vi "Update Contingency (SubVI).vi"(0 "array 1":i32[](array[numeric]), 1 "array 2":i32[](array[numeric]), 2 "array 3":i32[](array[numeric]), 3 "array 4":i32[](array[numeric]), 4 "Refnum in":refnum<k20>) -> ()   [LabVIEW 2013]
uses:
  <vilib>/rvi/interface/common/niFpgaWaitOnOcc.vi
  <vilib>/Utility/error.llb/Error Cluster From Error Code.vi
  <vilib>/rvi/errors/niLvFpgaAdjustHostInterfaceError.vi
  <vilib>/rvi/interface/nirviReadWriteControl/nirviReadWriteControl.xnode
  NiFpgaLv.dll
  <vilib>/rvi/interface/Simulation/niFpgaSimulationCallBeginRW.vi
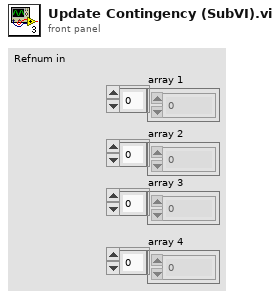
[diagram p1: front panel]
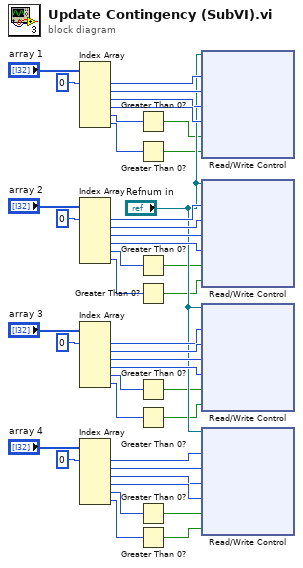
[diagram p0: block diagram]
diagram:
  n1 = Index Array(array="array 1", index #1=0 ("index")) -> (element #1=w26:i32, element #2=w27:i32, element #3=w28:i32, element #4=w29:i32, element #5=w14:i32, element #6=w13:i32)  [unwired: 5 in]
  n2 = Index Array(array="array 2", index #1=0 ("index")) -> (element #1=w41:i32, element #2=w40:i32, element #3=w39:i32, element #4=w38:i32, element #5=w10:i32, element #6=w9:i32)  [unwired: 5 in]
  n3 = Index Array(array="array 3", index #1=0 ("index")) -> (element #1=w34:i32, element #2=w35:i32, element #3=w36:i32, element #4=w37:i32, element #5=w6:i32, element #6=w5:i32)  [unwired: 5 in]
  n4 = Index Array(array="array 4", index #1=0 ("index")) -> (element #1=w30:i32, element #2=w31:i32, element #3=w32:i32, element #4=w33:i32, element #5=w2:i32, element #6=w1:i32)  [unwired: 5 in]
  n5 = Greater Than 0?(x=w14) -> (x > 0?=w15:bool)
  n6 = Greater Than 0?(x=w13) -> (x > 0?=w16:bool)
  n7 = Greater Than 0?(x=w10) -> (x > 0?=w11:bool)
  n8 = Greater Than 0?(x=w9) -> (x > 0?=w12:bool)
  n9 = Greater Than 0?(x=w6) -> (x > 0?=w8:bool)
  n10 = Greater Than 0?(x=w5) -> (x > 0?=w7:bool)
  n11 = Greater Than 0?(x=w2) -> (x > 0?=w3:bool)
  n12 = Greater Than 0?(x=w1) -> (x > 0?=w4:bool)
  n13 = xnode "Read/Write Control"("FPGA VI Reference In"="Refnum in", "Min Angle 1"=w26, "Max Angle 1"=w27, "Min Angle 1 2"=w28, "Max Angle 1 2"=w29, "CCW(T) 1"=w15, "CCW(T) 1 2"=w16) -> ()  [unwired: 1 in, 2 out]
  n14 = xnode "Read/Write Control"("FPGA VI Reference In"="Refnum in", "Min Angle 2"=w41, "Max Angle 2"=w40, "Min Angle 2 2"=w39, "Max Angle 2 2"=w38, "CCW(T)  2"=w11, "CCW(T)  2 2"=w12) -> ()  [unwired: 1 in, 2 out]
  n15 = xnode "Read/Write Control"("FPGA VI Reference In"="Refnum in", "Min Angle 3"=w34, "Max Angle 3"=w35, "Min Angle 3 2"=w36, "Max Angle 3 2"=w37, "CCW(T)  3"=w8, "CCW(T)  3 2"=w7) -> ()  [unwired: 1 in, 2 out]
  n16 = xnode "Read/Write Control"("FPGA VI Reference In"="Refnum in", "Min Angle 4"=w30, "Max Angle 4"=w31, "Min Angle 4 2"=w32, "Max Angle 4 2"=w33, "CCW(T)  4"=w3, "CCW(T)  4 2"=w4) -> ()  [unwired: 1 in, 2 out]
